vi "Eagle LinScale To Log.vi"(6 "MinScaleOut":dbl, 8 "MaxScaleOut":dbl, 9 "MinScaleIn":dbl, 10 "MaxScaleIn":dbl, 11 "ValIn":dbl) -> (3 "ValOut":dbl)   [LabVIEW 2015]
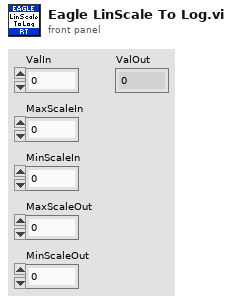
[diagram p1: front panel]
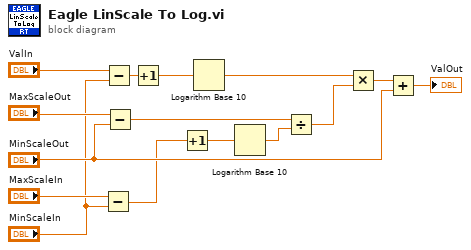
[diagram p0: block diagram]
diagram:
  n1 = Subtract(x="MaxScaleIn", y="MinScaleIn") -> (x-y=w10:dbl)
  n2 = Subtract(x="ValIn", y="MinScaleIn") -> (x-y=w7:dbl)
  n3 = Subtract(x="MaxScaleOut", y="MinScaleOut") -> (x-y=w13:dbl)
  n4 = Increment(x=w7) -> (x+1=w3:dbl)
  n5 = Increment(x=w10) -> (x+1=w2:dbl)
  n6 = Logarithm Base 10(1:w3) -> (0:w4:dbl)
  n7 = Logarithm Base 10(1:w2) -> (0:w1:dbl)
  n8 = Divide(x=w13, y=w1) -> (x/y=w12:dbl)
  n9 = Multiply(x=w4, y=w12) -> (x*y=w8:dbl)
  n10 = Add(x=w8, y="MinScaleOut") -> (x+y=→"ValOut":dbl)
